vi "Insert Format Code.vi"(8 "error in (no error)":errorcluster, 11 "Numeric Data Type in":refnum<class "Numeric Data Type.lvclass">) -> (0 "error out":errorcluster, 3 "Numeric Data Type (dup)":refnum<class "Numeric Data Type.lvclass">)   [LabVIEW 2018, in "Numeric Data Type.lvclass"]
uses:
  Numeric Data Type.lvclass
  Reference Format Codes.vi
  Reference Format String.vi
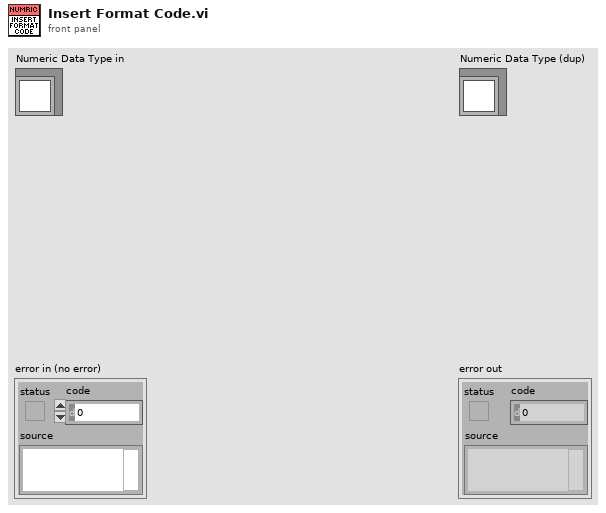
[diagram p1: front panel]
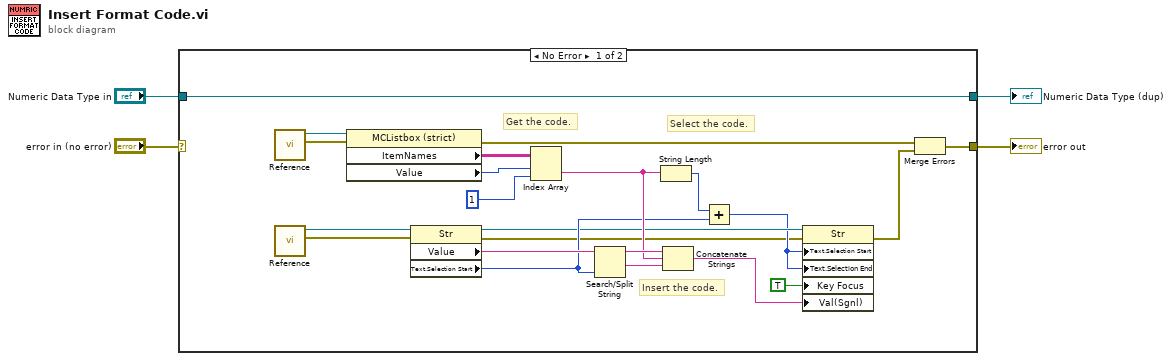
[diagram p0: block diagram]
diagram:
  n1 = case shown="No Error" "error in (no error)" {
    selector: "error in (no error)" -> [_ w28]
    tunnel: [w6 w28] -> w3
    tunnel: [w26 w27] -> w1
    tunnel: "Numeric Data Type in" -> [w26 w27]
    frame No Error {
      # "Get the code."
      # "Select the code."
      # "Insert the code."
      n2 = call-poly "Reference.vi"() -> ("error out"=w20:errorcluster, "Format Codes"=w25:refnum<vi>)  [unwired: 10 in]
      n3 = call-poly "Reference.vi"() -> ("error out"=w19:errorcluster, "Format String"=w21:refnum<vi>)  [unwired: 10 in]
      n4 = property class="MCListbox (strict)"(reference=w25, error in=w20) -> (error out=w7:errorcluster, "ItemNames"=w24:string[][], "Value"=w23:i32)  [unwired: 1 out]
      n5 = property class="Str"(reference=w21, error in=w19) -> (reference out=w12:refnum<vi>, error out=w8:errorcluster, "Value"=w14:string, "Text.Selection Start"=w13:u32)
      n6 = Index Array(array=w24, index (row)=w23, index (col)=1 ("disabled index (col)")) -> (element=w15:string)
      n7 = Search/Split String(string=w14, offset (0)=w13) -> (substring before match=w16:string, match + rest of string=w17:string)  [unwired: 2 out]
      n8 = String Length(string=w15) -> (length=w18:i32)
      n9 = Concatenate Strings(w16, w15, w17) -> (w9:string)
      n10 = Add(x=w18, y=w13) -> (x+y=w11:u32)
      n11 = property class="Str"(reference=w12, error in=w8, "Text.Selection Start"=w11, "Text.Selection End"=w11, "Key Focus"=TRUE, "Val(Sgnl)"=w9) -> (error out=w5:errorcluster)  [unwired: 1 out]
      n12 = Merge Errors(w7, w5) -> (w6:errorcluster)
    }
    frame Error {
    }
  }
  "error out" <- w3
  "Numeric Data Type (dup)" <- w1
